vi "Set MessageQ.vi"(10 "MessageQ":refnum<queue>, 11 "CD_Process in":refnum<class "Process.lvclass">) -> (3 "CD_Process out":refnum<class "Process.lvclass">)   [LabVIEW 2019, in "TimingDRV Engine.lvlib" / "Process.lvclass"]
uses:
  Process.lvclass
  TypeDefs/Message.ctl
  Process.lvclass/Process.ctl
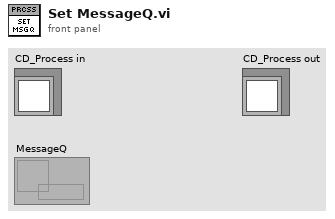
[diagram p1: front panel]
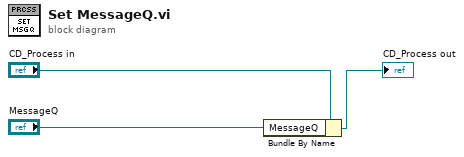
[diagram p0: block diagram]
diagram:
  n1 = Bundle By Name(cluster="CD_Process in", "MessageQ"="MessageQ") -> (→"CD_Process out":refnum<class "Process.lvclass">)
